vi "Configure XY Graph.vi"(4 "y name":string="A y name", 6 "x name":string="B x name", 7 "recolor traces?":bool, 8 "error in (no error)":errorcluster, 10 "XY Data []":cluster{"data":dbl[], "data":dbl[]}[](array[cluster]), 11 "XYGraph in":refnum<vi>) -> (0 "error out":errorcluster)   [LabVIEW 2016, in "Data.ITX.lvclass"]
uses:
  Data.ITX.lvclass
  <userlib>/LevyLab/Graph Utilities/graph_utilities.lvclass/graph_utilities.ctl
  <userlib>/LevyLab/Graph Utilities/graph_utilities.lvclass
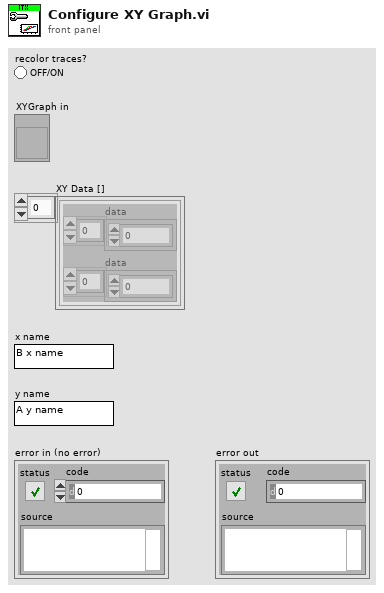
[diagram p1: front panel]
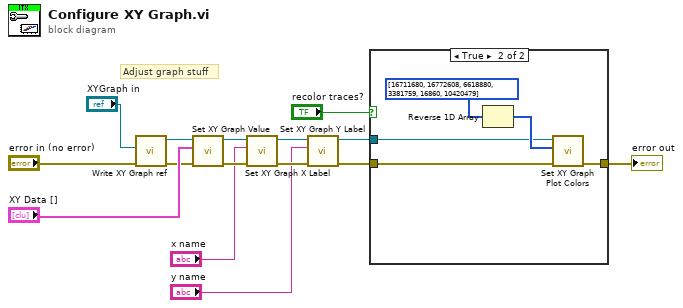
[diagram p0: block diagram]
diagram:
  # "Adjust graph stuff"
  n1 = call <userlib>:"Write XY Graph ref.vi"("error in (no error)"="error in (no error)", "XY Graph"="XYGraph in") -> ("error out"=w3:errorcluster, "graph_utilities out"=w7:refnum<class "graph_utilities.lvclass">)  [unwired: 8 in]
  n2 = call <userlib>:"Set XY Graph Value.vi"("error in (no error)"=w3, "Value"="XY Data []", "graph_utilities in"=w7) -> ("error out"=w9:errorcluster, "graph_utilities out"=w8:refnum<class "graph_utilities.lvclass">)  [unwired: 7 in]
  n3 = call <userlib>:"Set XY Graph X Label.vi"("error in (no error)"=w9, "X Label"="x name", "graph_utilities in"=w8) -> ("error out"=w11:errorcluster, "graph_utilities out"=w10:refnum<class "graph_utilities.lvclass">)  [unwired: 7 in]
  n4 = call <userlib>:"Set XY Graph Y Label.vi"("error in (no error)"=w11, "Y Label"="y name", "graph_utilities in"=w10) -> ("error out"=w14:errorcluster, "graph_utilities out"=w13:refnum<class "graph_utilities.lvclass">)  [unwired: 7 in]
  n5 = case shown="True" "recolor traces?" {
    tunnel: w13 -> [_ w20]
    tunnel: w14 -> [w16 w19]
    tunnel: [w16 w17] -> w1
    frame False {
    }
    frame True {
      n6 = Reverse 1D Array(array=u32[] [16711680, 16772608, 6618880, 3381759, 16860, 10420479] ("color scale")) -> (reversed array=w21:u32[])
      n7 = call <userlib>:"Set XY Graph Plot Colors.vi"("error in (no error)"=w19, "Colors []"=w21, "graph_utilities in"=w20) -> ("error out"=w17:errorcluster)  [unwired: 7 in, 1 out]
    }
  }
  "error out" <- w1
